vi "matrici_v41.vi"() -> ()   [LabVIEW 2009]
uses:
  <vilib>/Math Plots/3D Math Plots/3D Surface/3D Surface XCtrl/3D Surface.xctl
  <vilib>/Math Plots/3D Math Plots/3D Surface/3D Surface Datatype/3D Surface Datatype.lvclass
  <vilib>/Math Plots/3D Math Plots/3D Surface/3D Surface Datatype/Public/Plot Helper (Vector).vi
panel:
  out "X":dbl=2.000000000000001
  out "y":dbl=2.000000000000001
  in  "Rezolutia":dbl(slide)=28.67132867132867 scale=10.0..100.0
  in  "stop":bool
  out "3D Surface":refnum<class "3D Plot Datatype.lvclass">[](xcontrol)
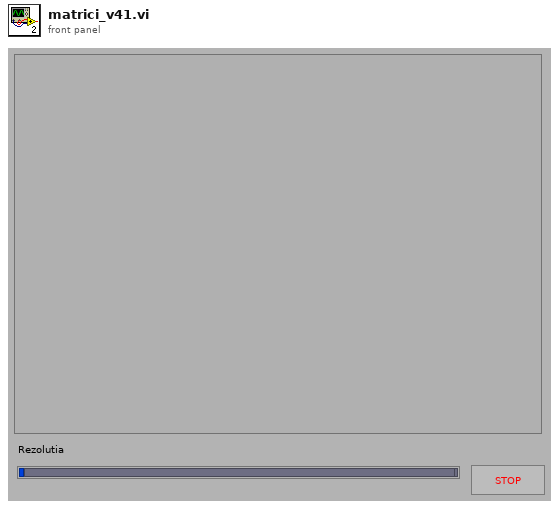
[diagram p1: front panel]
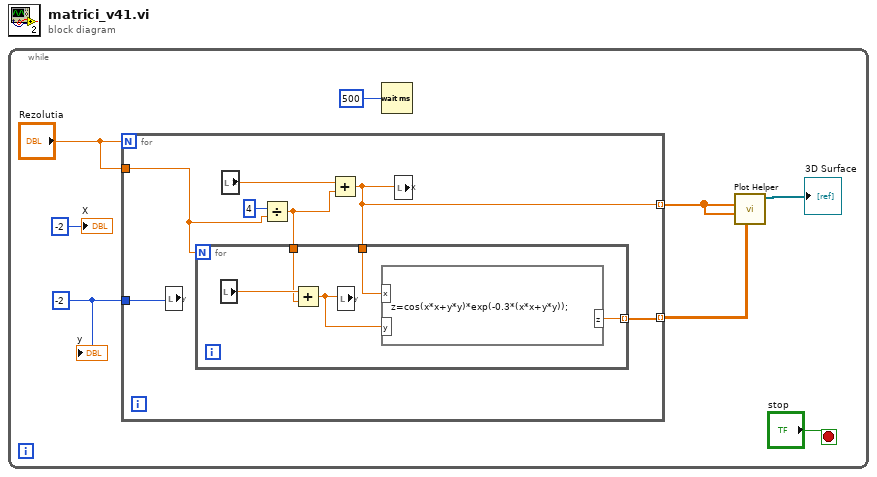
[diagram p0: block diagram]
diagram:
  n1 = while {
    stop <- "stop" stop-if-true
    w5 = -2
    n2 = for {
      N: "Rezolutia" -> [_]
      tunnel: [w14] -> w6 mode=indexing
      tunnel: [w13] -> w1 mode=indexing
      tunnel: "Rezolutia" -> [w11]
      tunnel: w5 -> [w9]
      n3 = local write "y"(w9) -> ()
      n4 = local read "X"() -> (w15:dbl)
      n5 = Divide(x=4, y=w11) -> (x/y=w10:dbl)
      n6 = Add(x=w15, y=w10) -> (x+y=w14:dbl)
      n7 = for {
        N: w11 -> [_]
        tunnel: w14 -> [w19]
        tunnel: [w17] -> w13 mode=indexing
        tunnel: w10 -> [w16]
        n8 = local read "y"() -> (w20:dbl)
        n9 = Add(x=w20, y=w16) -> (x+y=w18:dbl)
        n10 = local write "y"(w18) -> ()
        n11 = formula code="z=cos(x*x+y*y)*exp(-0.3*(x*x+y*y));"("x"=w19, "y"=w18) -> ("z"=w17:dbl)
      }
      n12 = local write "X"(w14) -> ()
    }
    n13 = Wait (ms)(milliseconds to wait=500) -> ()  [unwired: 1 out]
    n14 = call-poly <vilib>:"Plot Helper.vi"("z matrix"=w1, "y vector"=w6, "x vector"=w6) -> ("3D Plot lvclass Array out"=→"3D Surface":refnum<class "3D Plot Datatype.lvclass">[])  [unwired: 3 in, 5 out]
    "X" <- -2
    "y" <- w5
  }
